vi "GetMethod.vi"(6 "CommandVI":string, 9 "CallMode":T1, 11 "ReferencesIn":variant[](array[variant])) -> (0 "ErrorOut":errorcluster, 2 "VIOut":refnum<vi>, 3 "ReferencesOut":variant[](array[variant]))   [LabVIEW 2021, in "YActor.lvclass"]
uses:
  YActor.lvclass
  CallMode.ctl
  VIMethodTemplate.vi
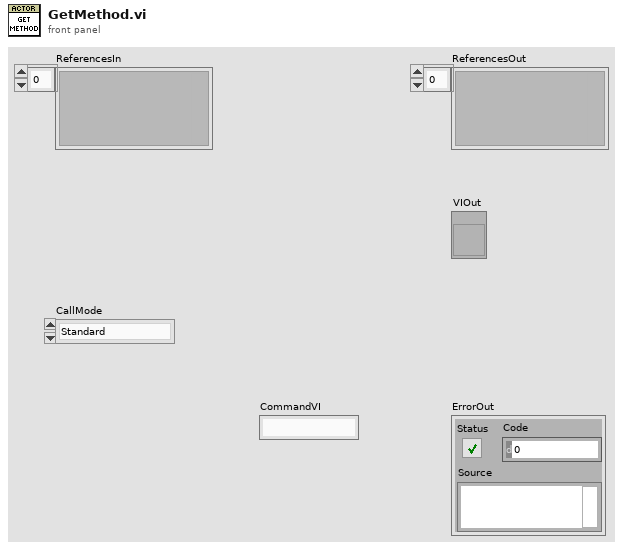
[diagram p1: front panel]
types:
  T1 = typedef "YActor.lvclass/CallMode.ctl" = enum16{"Standard", "Call&Collect"}
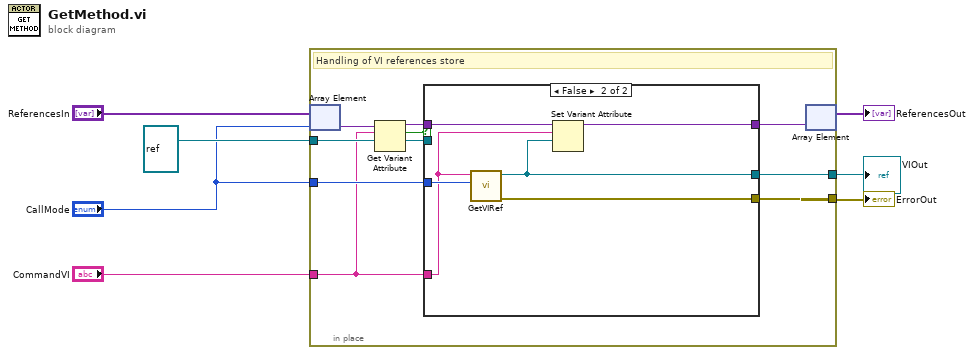
[diagram p0: block diagram]
diagram:
  n1 = in-place {
    in-place-border: [w16] -> w1
    in-place-border: [w17] -> w7
    in-place-border: "CommandVI" -> [w12]
    in-place-border: "CallMode" -> [w15]
    in-place-border: refnum<vi> refnum ("VI in") -> [w13]
    # "Handling of VI references store"
    n2 = in-place-array #1("ReferencesIn", "CallMode") -> (w14:variant)
    n3 = Get Variant Attribute(Variant=w14, name=w12, default value (empty Variant)=w13) -> (duplicate Variant=w9:variant, found=w11:bool, value=w10:refnum<vi>)  [unwired: 1 in, 1 out]
    n4 = case shown="False" w11 {
      tunnel: w12 -> [_ w22]
      tunnel: [w19 w21] -> w16
      tunnel: [_ w25] -> w17
      tunnel: w15 -> [_ w24]
      tunnel: w10 -> [w19 _]
      tunnel: w9 -> [w18 w23]
      tunnel: [w18 w20] -> w8
      frame True {
      }
      frame False {
        n5 = call "GetVIRef.vi"("CallMode"=w24, "CommandVI"=w22) -> ("ErrorOut"=w25:errorcluster, "VIOut"=w21:refnum<vi>)  [unwired: 8 in]
        n6 = Set Variant Attribute(Variant=w23, name=w22, value=w21) -> (Variant out=w20:variant)  [unwired: 1 in, 2 out]
      }
    }
    n7 = in-place-array #1(w8) -> (→"ReferencesOut":variant[])  [unwired: 1 out]
  }
  "ErrorOut" <- w7
  "VIOut" <- w1
